vi "receiveILCData.vi"(8 "error in (no error)":errorcluster, 11 "Model in":refnum<class "Model.lvclass">) -> (0 "error out":errorcluster, 3 "Model out":refnum<class "Model.lvclass">)   [LabVIEW 2013, in "Model.lvclass"]
uses:
  Model.lvclass
  Model.lvclass/Model.ctl
  UserEvents/UserEvents.lvclass/UserEvents.ctl
  ApplicationElements/Log/TestDataLog/TestDataLog.lvclass/TestDataLog.ctl
  <userlib>/Common/ILC/ILC/ILC.lvclass/ILC.ctl
  <userlib>/Common/ILC/ILC/ILC.lvclass
  UserEvents/UserEvents.lvclass
  ApplicationElements/Log/TestDataLog/TestDataLog.lvclass
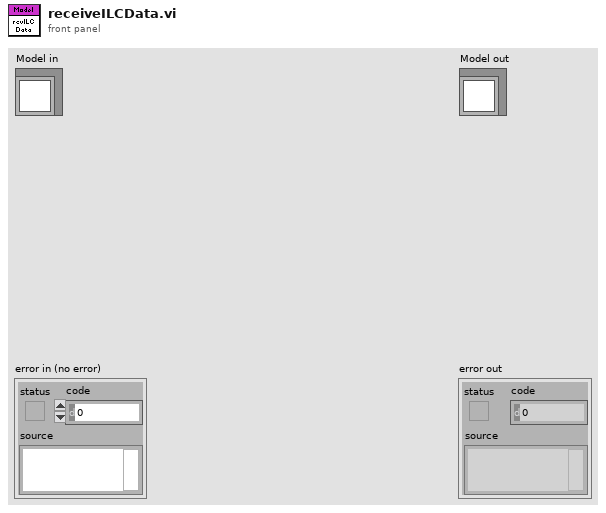
[diagram p1: front panel]
types:
  T1 = typedef "AITDTTypedefs.lvlib/InputData.ctl" = cluster{"Temperature Measured":dbl[unit], "ADCs":T2}
  T2 = typedef "ILCCommon.lvlib/ILCTypedefs.lvlib/ADCs.ctl" = cluster{"Ch0":i32, "Ch1":i32, "Ch2":i32, "Ch3":i32, "Ch4":i32}
  T3 = typedef "ILCCommon.lvlib/ILCTypedefs.lvlib/ADCsInEngineeringUnits.ctl" = cluster{"Ch1":dbl[unit], "Ch2":dbl[unit], "Ch3":dbl[unit], "Ch4":dbl[unit]}
  T4 = typedef "ILCCommon.lvlib/ILCTypedefs.lvlib/InputData.ctl" = cluster{"Input Channels":T5, "Limit Switches":T6, "Tachometer":u16, "SSI Encoder":i32, "ADCs":T2}
  T5 = typedef "ILCCommon.lvlib/ILCConfiguration.lvlib/InputChannels.ctl" = enum16{"Channel 0", "3 Channels", "5 Channels"}
  T6 = typedef "ILCCommon.lvlib/ILCTypedefs.lvlib/LimitSwitches.ctl" = cluster{"1":bool, "2":bool}
  T7 = typedef "AITDTTypedefs.lvlib/PubDataEvents.ctl" = cluster{"State":refnum<user-event>, "ErrorCode":refnum<user-event>, "OutputData":refnum<user-event>, "InputData":refnum<user-event>, "TestStatus":refnum<user-event>, "LogPath":refnum<user-event>, "TemperatureSetpointRequest":refnum<user-event>, "TemperatureSettling":refnum<user-event>, "WaitTimeStatus":refnum<user-event>}
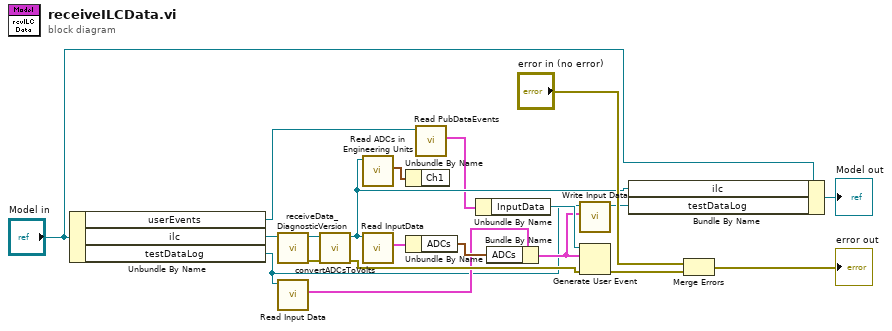
[diagram p0: block diagram]
diagram:
  n1 = Unbundle By Name("Model in") -> ("userEvents"=w9:refnum<class "UserEvents.lvclass">, "ilc"=w5:refnum<class "ILC.lvclass">, "testDataLog"=w1:refnum<class "TestDataLog.lvclass">)
  n2 = call <userlib>:"receiveData_DiagnosticVersion.vi"("ILC in"=w5) -> ("error out"=w14:errorcluster, "ILC out"=w15:refnum<class "ILC.lvclass">)  [unwired: 9 in]
  n3 = call "Read Input Data.vi"("TestDataLog in"=w1) -> ("Input Data"=w2:T1)  [unwired: 9 in, 1 out]
  n4 = call <userlib>:"convertADCsToVolts.vi"("error in (no error)"=w14, "ILC in"=w15) -> ("error out"=w13:errorcluster, "ILC out"=w8:refnum<class "ILC.lvclass">)  [unwired: 8 in]
  n5 = call <userlib>:"Read ADCs in Engineering Units.vi"("ILC in"=w8) -> ("ADCs in Engineering Units"=w12:T3)  [unwired: 9 in, 1 out]
  n6 = call <userlib>:"Read InputData.vi"("ILC in"=w8) -> ("InputData"=w4:T4)  [unwired: 9 in, 1 out]
  n7 = Unbundle By Name(w12) -> ()  [unwired: 1 out]
  n8 = Unbundle By Name(w4) -> ("ADCs"=w3:T2)
  n9 = call "Read PubDataEvents.vi"("UserEvents in"=w9) -> ("PubDataEvents"=w6:T7)  [unwired: 9 in, 1 out]
  n10 = Unbundle By Name(w6) -> ("InputData"=w10:refnum<user-event>)
  n11 = Bundle By Name(cluster=w2, "ADCs"=w3) -> (w7:T1)
  n12 = call "Write Input Data.vi"("Input Data"=w7, "Logger in"=w1) -> ("Logger out"=w11:refnum<class "TestDataLog.lvclass">)  [unwired: 9 in]
  n13 = Generate User Event(user event=w10, event data cluster=w7, error in=w13) -> (error out=w17:errorcluster)  [unwired: 1 in, 1 out]
  n14 = Bundle By Name(cluster="Model in", "ilc"=w8, "testDataLog"=w11) -> (→"Model out":refnum<class "Model.lvclass">)
  n15 = Merge Errors("error in (no error)", w17) -> (→"error out":errorcluster)
